vi "Unflatten String.vi"(11 "Tag value":string) -> (3 "String":string)   [LabVIEW 2020, in "NI_VIAn_XML Parsing.lvlib"]
uses:
  <vilib>/addons/analyzer/XML Parsing/NI_VIAn_XML Parsing.lvlib
  <vilib>/addons/analyzer/VIAnCFGDataStructure/Tree Manager/API/Generate Hash.vi
  <vilib>/addons/analyzer/VIAnCFGDataStructure/Tree Manager/Tree.lvclass
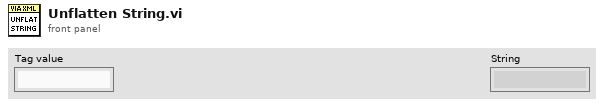
[diagram p1: front panel]
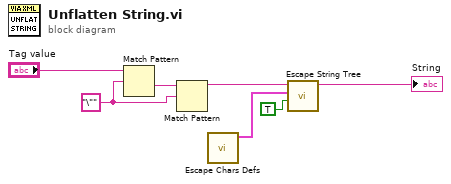
[diagram p0: block diagram]
diagram:
  w6 = "\"" ("regular expression")
  n1 = Match Pattern(string="Tag value", regular expression=w6) -> (after substring=w5:string)  [unwired: 1 in, 3 out]
  n2 = Match Pattern(string=w5, regular expression=w6) -> (before substring=w2:string)  [unwired: 1 in, 3 out]
  n3 = call <vilib>:"Escape Chars Defs.vi"() -> ("Escapes"=w3:cluster{"String":string, "Escape":string}[])  [unwired: 11 in]
  n4 = call <vilib>:"Escape String Tree.vi"("Reverse? (False)"=TRUE, "Escapes"=w3, "String In"=w2) -> ("String Out"=→"String":string)  [unwired: 8 in]
